vi "Lab 2b.vi"() -> ()   [LabVIEW 2011]
uses:
  subVIs_Dcomm_offered/FilterCoefficient.ctl
panel:
  in  "filter parameters":T1={"Alpha"=0.5, "Filter Length"=6, "TX Filter"=enum."Root Raised Cos"} {"Alpha" format="%.2f"}
  out "Calculated BER":dbl[](array[numeric])
  out "BER":cluster{"Y":dbl[], "Y":dbl[]}[](graph)
  in  "SNR [dB]":dbl[](array[numeric])
  in  "Mapping Parameters":T2={"Modulation Order"=2, "Modulation Type"=0, "Samples per Symbol"=8} {"Modulation Type" items=["PSK", "QAM"]}
  in  "Mapping Parameters":T2={"Modulation Order"=2, "Modulation Type"=0, "Samples per Symbol"=8} {"Modulation Type" items=["PSK", "QAM"]}
  in  "Mapping Parameters":T2={"Modulation Order"=2, "Modulation Type"=0, "Samples per Symbol"=8} {"Modulation Type" items=["PSK", "QAM"]}
  in  "Mapping Parameters":T2={"Modulation Order"=2, "Modulation Type"=0, "Samples per Symbol"=8} {"Modulation Type" items=["PSK", "QAM"]}
  in  "Choose the Format":enum32{"BPSK", "QPSK", "16QAM", "64QAM"}(tab)
  in  "System Parameters":T3={"Samples per Symbol"=8, "symbol map"=[]} {"symbol map" format="%.3f"}
  in  "System Parameters":T3={"Samples per Symbol"=8, "symbol map"=[]} {"symbol map" format="%.3f"}
  in  "System Parameters":T3={"Samples per Symbol"=8, "symbol map"=[]} {"symbol map" format="%.3f"}
  in  "System Parameters":T3={"Samples per Symbol"=8, "symbol map"=[]} {"symbol map" format="%.3f"}
  in  "Num of Symbols":i32=100
  # "Lab 2(b) Digital Communication with LabVIEW"
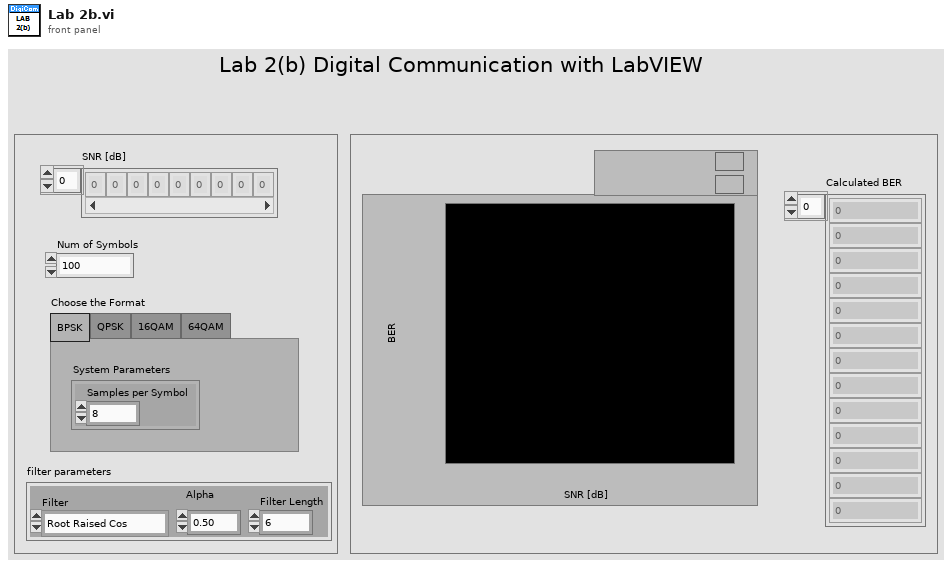
[diagram p1: front panel]
types:
  T1 = typedef "FilterCoefficient.ctl" = cluster{"Alpha":dbl, "Filter Length":i32, "TX Filter":enum16{"Root Raised Cos", "Raised Cos", "Rectangular"}}
  T2 = cluster{"Modulation Order":i32, "Modulation Type":u16, "Samples per Symbol":i32}
  T3 = cluster{"Samples per Symbol":i32, "symbol map":cdb[]}
  T4 = typedef "niAMT.lvlib/Complex Data Waveform.ctl" = cluster{"t0":dbl, "dt":dbl, "Y":cdb[]}
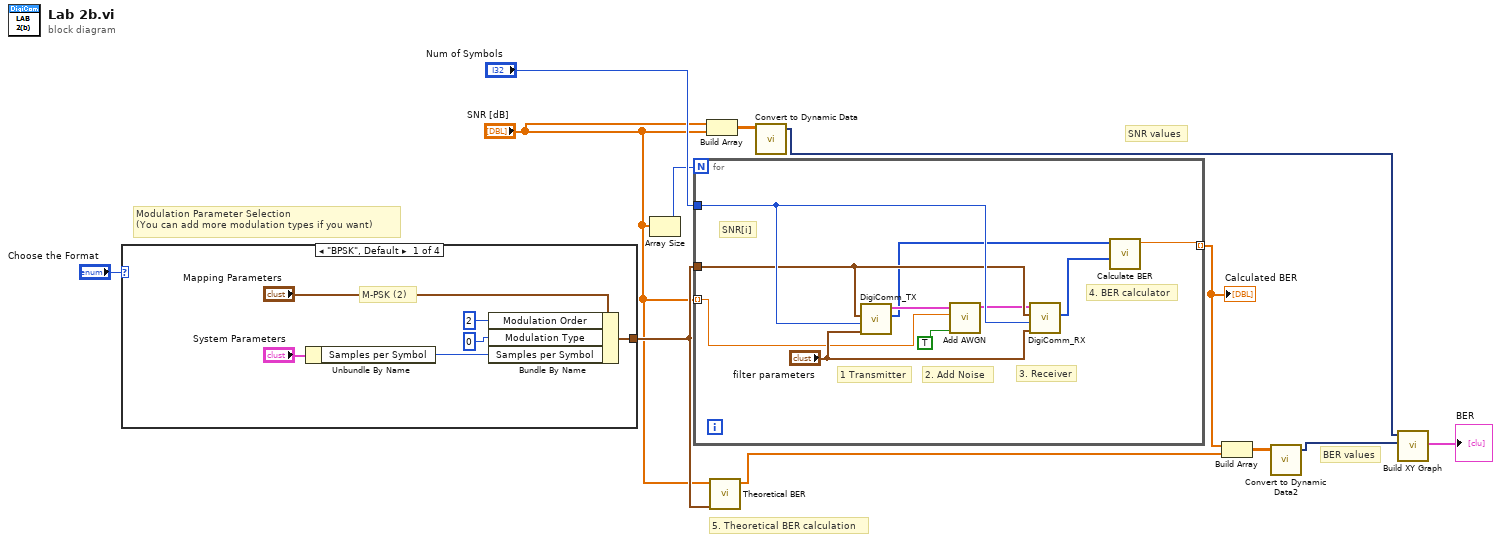
[diagram p0: block diagram]
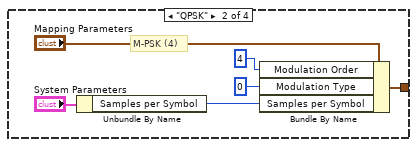
[diagram p2: hidden frame]
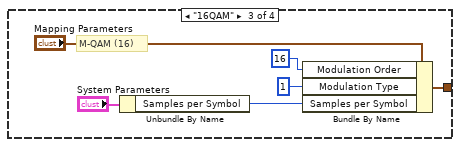
[diagram p3: hidden frame]
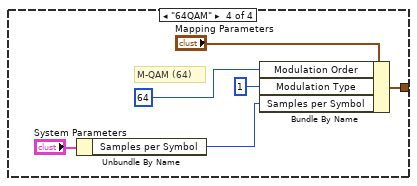
[diagram p4: hidden frame]
diagram:
  # "5. Theoretical BER calculation"
  # "BER values"
  # "SNR values"
  # "Modulation Parameter Selection\n(You can add more modulation types if you want)"
  n1 = case shown="\"BPSK\", Default" "Choose the Format" {
    tunnel: [w13 w21 w25 w31] -> w9
    frame "BPSK", Default {
      # "M-PSK (2)"
      n2 = Unbundle By Name("System Parameters") -> ("Samples per Symbol"=w14:i32)
      n3 = Bundle By Name(cluster="Mapping Parameters", "Modulation Order"=2, "Modulation Type"=u16 0, "Samples per Symbol"=w14) -> (w13:T2)
    }
    frame "QPSK" {
      # "M-PSK (4)"
      n4 = Unbundle By Name("System Parameters") -> ("Samples per Symbol"=w19:i32)
      n5 = Bundle By Name(cluster="Mapping Parameters", "Modulation Order"=4, "Modulation Type"=u16 0, "Samples per Symbol"=w19) -> (w21:T2)
    }
    frame "16QAM" {
      # "M-QAM (16)"
      n6 = Unbundle By Name("System Parameters") -> ("Samples per Symbol"=w26:i32)
      n7 = Bundle By Name(cluster="Mapping Parameters", "Modulation Order"=16, "Modulation Type"=u16 1, "Samples per Symbol"=w26) -> (w25:T2)
    }
    frame "64QAM" {
      # "M-QAM (64)"
      n8 = Unbundle By Name("System Parameters") -> ("Samples per Symbol"=w32:i32)
      n9 = Bundle By Name(cluster="Mapping Parameters", "Modulation Order"=64, "Modulation Type"=u16 1, "Samples per Symbol"=w32) -> (w31:T2)
    }
  }
  n10 = Array Size(array="SNR [dB]") -> (size(s)=w2:i32)
  n11 = for {
    N: w2 -> [_]
    tunnel: w9 -> [w42]
    tunnel: "SNR [dB]" -> [w38] mode=indexing
    tunnel: [w45] -> w10 mode=indexing
    tunnel: "Num of Symbols" -> [w44]
    # "4. BER calculator"
    # "3. Receiver"
    # "2. Add Noise"
    # "1 Transmitter"
    # "SNR[i]"
    n12 = call "DigiComm_TX.vi"("filter parameters"="filter parameters", "Num of Symbols"=w44, "Mapping Parameters"=w42) -> ("input bit stream"=w40:i16[], "input complex waveform"=w46:T4)  [unwired: 5 in]
    n13 = call "Add AWGN.vi"("Add AWGN?"=TRUE, "SNR [dB]"=w38, "Input"=w46) -> ("Output"=w37:cluster{"t0":dbl, "dt":dbl, "Y":cdb[]})  [unwired: 8 in]
    n14 = call "DigiComm_RX.vi"("filter parameters"="filter parameters", "Number of Symbols"=w44, "Mapping Parameters"=w42, "data waveform"=w37) -> ("Output Bit Stream"=w43:i8[])  [unwired: 6 in]
    n15 = call "Calculate BER.vi"("Output Stream"=w43, "Input Stream"=w40) -> ("BER"=w45:dbl)  [unwired: 9 in]
  }
  "Calculated BER" <- w10
  n16 = Build Array("SNR [dB]", "SNR [dB]") -> (w7:dbl[][])
  n17 = call "Theoretical BER.vi"("Mapping Parameters"=w9, "SNRdB"="SNR [dB]") -> ("BER"=w8:dbl[])  [unwired: 9 in]
  n18 = call "Convert to Dynamic Data"("2D Array"=w7) -> ("Dynamic Data Type"=w6:dynamicdata)  [unwired: 3 in]
  n19 = Build Array(w10, w8) -> (w5:dbl[][])
  n20 = call "Convert to Dynamic Data2"("2D Array"=w5) -> ("Dynamic Data Type"=w4:dynamicdata)  [unwired: 3 in]
  n21 = call "Build XY Graph"("Y Input"=w4, "X Input"=w6) -> ("XY Graph"=→"BER":cluster{"Y":dbl[], "Y":dbl[]}[])  [unwired: 3 in, 6 out]
